vi "Pump + UDP.vi"() -> ()   [LabVIEW 2018]
uses:
  Node 2 - States.ctl
  Shared/Globals.vi
panel:
  out "PUMP STATE":bool
  in  "stop":bool
  # "ON"
  # "OFF"
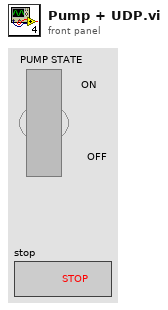
[diagram p1: front panel]
types:
  T1 = typedef "Node 2 - States.ctl" = enum16{"Initialize", "Read Pump State", "Toggle Pump", "Send HB", "Error"}
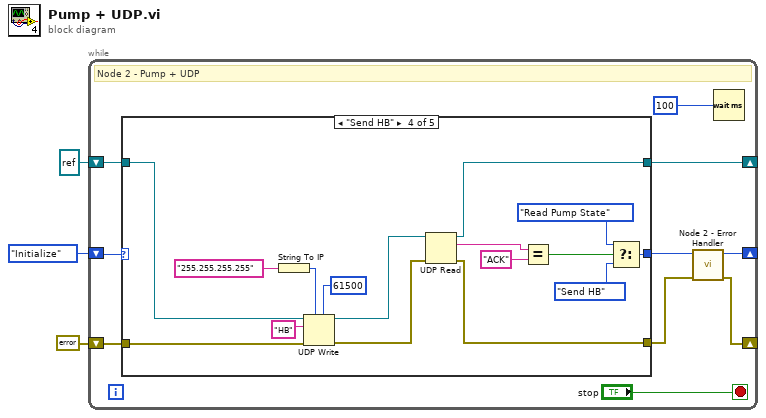
[diagram p0: block diagram]
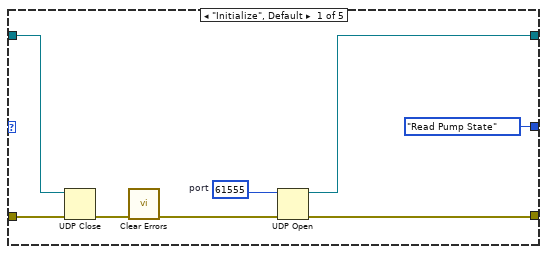
[diagram p2: hidden frame]
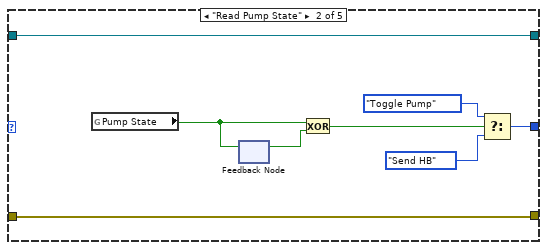
[diagram p3: hidden frame]
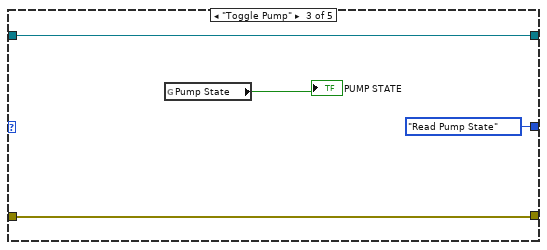
[diagram p4: hidden frame]
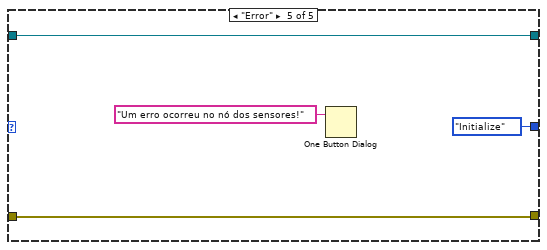
[diagram p5: hidden frame]
diagram:
  n1 = while {
    shift-right: [w9] -> _
    shift-left: Node_2_-_States."Initialize" -> [w12]
    shift-right: [w8] -> _
    shift-left: errorcluster {"status"=FALSE, "code"=0, "source"=""} ("Error Out") -> [w6]
    shift-right: [w5] -> _
    shift-left: refnum<k16> refnum ("connection ID out") -> [w4]
    stop <- "stop" stop-if-true
    # "Node 2 - Pump + UDP"
    n2 = case shown="\"Send HB\"" w12 {
      tunnel: [Node_2_-_States."Read Pump State" w27 Node_2_-_States."Read Pump State" w49 Node_2_-_States."Initialize"] -> w11
      tunnel: [w15 w23 w31 w34 w52] -> w7
      tunnel: w6 -> [w14 w23 w31 w42 w52]
      tunnel: [w19 w22 w30 w41 w50] -> w5
      tunnel: w4 -> [w17 w22 w30 w48 w50]
      frame "Initialize", Default {
        w20 = u16 61555  # port
        n3 = UDP Close(connection ID=w17, 8:w14) -> (error out=w18:errorcluster)  [unwired: 1 out]
        n4 = call <vilib>:"Clear Errors.vi"("error in (no error)"=w18) -> ("error out"=w16:errorcluster)  [unwired: 5 in, 1 out]
        n5 = UDP Open(8:w16, 11:w20) -> (port=w19:refnum<k16>, 0:w15:errorcluster)  [unwired: 3 in, 1 out]
      }
      frame "Read Pump State" {
        n6 = global read "Globals.vi" "Pump State"() -> (w24:bool)
        n7 = feedback-in #1(w24) -> ()
        n8 = feedback #1() -> (w26:bool)  [unwired: 1 in]
        n9 = Exclusive Or(1:w26, 2:w24) -> (0:w25:bool)
        n10 = Select(t=Node_2_-_States."Toggle Pump", s=w25, f=Node_2_-_States."Send HB") -> (s? t:f=w27:T1)
      }
      frame "Toggle Pump" {
        n11 = global read "Globals.vi" "Pump State"() -> (→"PUMP STATE":bool)
      }
      frame "Send HB" {
        n12 = String To IP(1:"255.255.255.255") -> (0:w45:u32)
        n13 = UDP Write(address=w45, port or service name=u16 61500, connection ID=w48, data in="HB", 8:w42) -> (error out=w40:errorcluster, 3:w43:refnum<k16>)  [unwired: 1 in]
        n14 = UDP Read(connection ID=w43, 8:w40) -> (data out=w39:string, error out=w34:errorcluster, 3:w41:refnum<k16>)  [unwired: 2 in, 2 out]
        n15 = Equal?(x=w39, y="ACK") -> (x = y?=w35:bool)
        n16 = Select(t=Node_2_-_States."Read Pump State", s=w35, f=Node_2_-_States."Send HB") -> (s? t:f=w49:T1)
      }
      frame "Error" {
        n17 = One Button Dialog(message="Um erro ocorreu no nó dos sensores!") -> ()  [unwired: 1 in, 1 out]
      }
    }
    n18 = call "Node 2 - Error Handler.vi"("Error In"=w7, "State In"=w11) -> ("Error Out"=w8:errorcluster, "State Out"=w9:T1)  [unwired: 8 in]
    n19 = Wait (ms)(milliseconds to wait=u32 100) -> ()  [unwired: 1 out]
  }
